vi "Alternate BG Color.vi"(6 "Row Or Col":T1, 8 "错误输入":errorcluster, 9 "Second BG Color":u32(colorbox), 10 "First BG Color":u32(colorbox), 11 "Mlistbox Ref":refnum<vi>) -> (0 "错误输出":errorcluster, 3 "Mlistbox Ref Dup":refnum<vi>)   [LabVIEW 2012, in "Mlistbox Tools.lvlib"]
uses:
  Mlistbox Tools.lvlib
  Custom Type/Row and Col Option.ctl
  ListBox/Custom Type/Read and Write Mode.ctl
  Property/Set and Get Num of Rows Or Cols.vi
  Property/Set and Get Active Cell BG Color.vi
  ListBox/Listbox Tool.lvlib
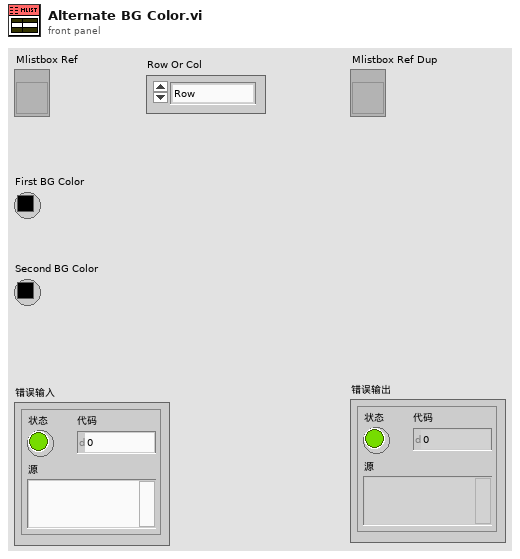
[diagram p1: front panel]
types:
  T1 = typedef "Mlistbox Tools.lvlib/Row and Col Option.ctl" = enum16{"Row", "Col"}
  T2 = typedef "Listbox Tool.lvlib/Read and Write Mode.ctl" = enum16{"Read", "Write"}
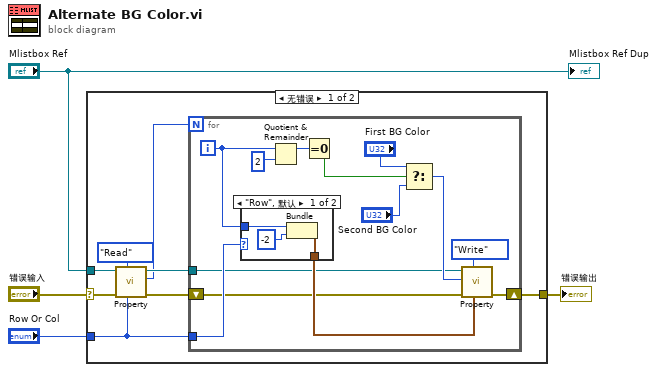
[diagram p0: block diagram]
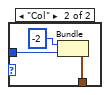
[diagram p2: hidden frame]
diagram:
  n1 = case shown="无错误" "错误输入" {
    selector: "错误输入" -> [w7 w32]
    tunnel: "Row Or Col" -> [w12 _]
    tunnel: [w6 w32] -> w2
    tunnel: "Mlistbox Ref" -> [w11 _]
    frame No Error {
      n2 = call-poly "Property.vi"("Row Or Col"=w12, "Mode"=Read_and_Write_Mode."Read", "错误输入"=w7, "Mlistbox Ref"=w11) -> ("错误输出"=w5:errorcluster, "Number of Rows or Cols Out"=w8:u32, "Mlistbox Ref Dup"=w9:refnum<vi>)  [unwired: 5 in]
      n3 = for {
        N: w8 -> [_]
        tunnel: w12 -> [w25]
        tunnel: w9 -> [w14]
        shift-right: [w24] -> w6
        shift-left: w5 -> [w13]
        i -> [w22]
        n4 = case shown="\"Row\", 默认" w25 {
          tunnel: w22 -> [w28 w31]
          tunnel: [w26 w29] -> w15
          frame "Row", Default {
            n5 = Bundle(w28, -2) -> (w26:cluster{i32, i32})  [unwired: 1 in]
          }
          frame "Col" {
            n6 = Bundle(-2, w31) -> (w29:cluster{i32, i32})  [unwired: 1 in]
          }
        }
        n7 = Quotient & Remainder(x=w22, y=2) -> (x-y*floor(x/y)=w20:i32)  [unwired: 1 out]
        n8 = Equal To 0?(x=w20) -> (x = 0?=w19:bool)
        n9 = Select(t="First BG Color", s=w19, f="Second BG Color") -> (s? t:f=w16:u32)
        n10 = call-poly "Property.vi"("Active Cell In"=w15, "Mode"=Read_and_Write_Mode."Write", "错误输入"=w13, "Active Cell BG Color In"=w16, "Mlistbox Ref"=w14) -> ("错误输出"=w24:errorcluster)  [unwired: 4 in, 2 out]
      }
    }
    frame Error {
    }
  }
  "错误输出" <- w2
  "Mlistbox Ref Dup" <- "Mlistbox Ref"
